vi "MassAverages.vi"(2 "Input Cluster":T3, 3 "N":dbl, 4 "Array In Cluster":T1) -> (0 "Average Cluster":T2, 1 "Array Out Cluster":T1)   [LabVIEW 2021]
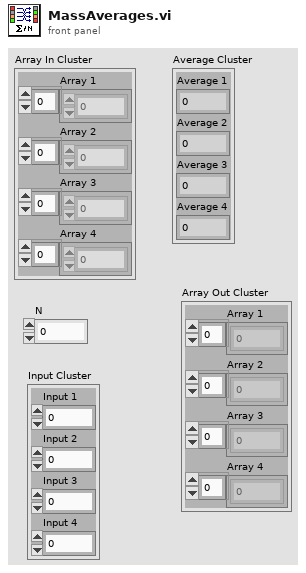
[diagram p1: front panel]
types:
  T1 = cluster{"Array 1":dbl[], "Array 2":dbl[], "Array 3":dbl[], "Array 4":dbl[]}
  T2 = cluster{"Average 1":dbl, "Average 2":dbl, "Average 3":dbl, "Average 4":dbl}
  T3 = cluster{"Input 1":dbl, "Input 2":dbl, "Input 3":dbl, "Input 4":dbl}
  T4 = cluster{"Average":dbl, "Average":dbl, "Average":dbl, "Average":dbl}
  T5 = cluster{"Array Out":dbl[], "Array Out":dbl[], "Array Out":dbl[], "Array Out":dbl[]}
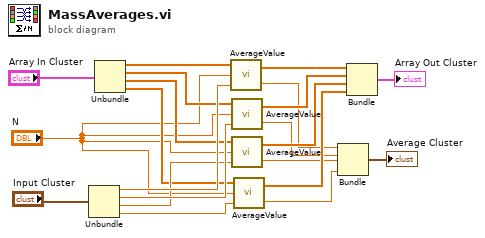
[diagram p0: block diagram]
diagram:
  n1 = Unbundle("Input Cluster") -> ("Input 1"=w18:dbl, "Input 2"=w16:dbl, "Input 3"=w14:dbl, "Input 4"=w12:dbl)
  n2 = Unbundle("Array In Cluster") -> ("Array 1"=w19:dbl[], "Array 2"=w17:dbl[], "Array 3"=w15:dbl[], "Array 4"=w13:dbl[])
  n3 = call "AverageValue.vi"("Running Input"=w18, "N"="N", "Array In"=w19) -> ("Average"=w6:dbl, "Array Out"=w11:dbl[])
  n4 = call "AverageValue.vi"("Running Input"=w16, "N"="N", "Array In"=w17) -> ("Average"=w5:dbl, "Array Out"=w10:dbl[])
  n5 = call "AverageValue.vi"("Running Input"=w14, "N"="N", "Array In"=w15) -> ("Average"=w4:dbl, "Array Out"=w9:dbl[])
  n6 = call "AverageValue.vi"("Running Input"=w12, "N"="N", "Array In"=w13) -> ("Average"=w3:dbl, "Array Out"=w8:dbl[])
  n7 = Bundle("Average"=w6, "Average"=w5, "Average"=w4, "Average"=w3) -> (→"Average Cluster":T4)  [unwired: 1 in]
  n8 = Bundle("Array Out"=w11, "Array Out"=w10, "Array Out"=w9, "Array Out"=w8) -> (→"Array Out Cluster":T5)  [unwired: 1 in]
